vi "arm control.vi"(1 "State":T1, 2 "Z Axis (Tuning)":dbl) -> (0 "setpoint":dbl format="%.2f")   [LabVIEW 2013]
uses:
  typedefs/subStates.ctl
  typedefs/fg_typedef.ctl
panel:
  in  "lower limit":dbl=-0.015 format="%#_13g"
  in  "upper limit":dbl=0.015 format="%#_13g"
  in  "Up Setpoint":dbl format="%#_13g"
  # "Things needing Tuning"
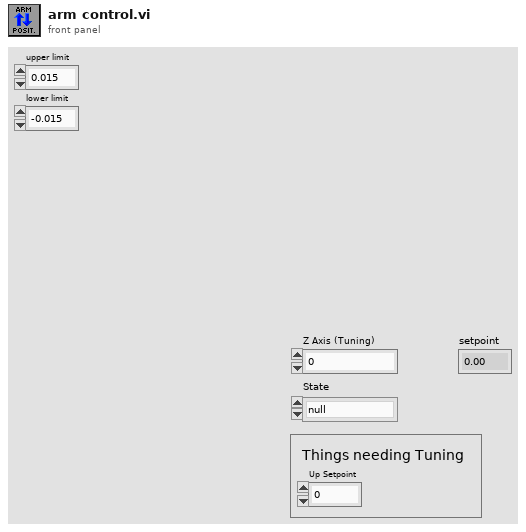
[diagram p1: front panel]
types:
  T1 = typedef "subStates.ctl" = enum16{"null", "wait", "driver control", "auto", "manual override", "hold position", "rotate", "pickup", "pass", "load", "goto shoot", "shoot", "cancel", "end"}
  T2 = typedef "fg_typedef.ctl" = enum16{"Get", "Set"}
  T3 = typedef "WPI_DigitalInputDevRef.ctl" = cluster{"DevStatus":errorcluster, "DIO Channel":T4, "Digital Module":T5}
  T4 = typedef "FPGA_DIOChannel.ctl" = enum8{"DIO 1", "DIO 2", "DIO 3", "DIO 4", "DIO 5", "DIO 6", "DIO 7", "DIO 8", "DIO 9", "DIO 10", "DIO 11", "DIO 12", "DIO 13", "DIO 14", "Invalid"}
  T5 = typedef "FPGA_TypedefDigitalModule.ctl" = enum16{"Digital Module 1", "Digital Module 2"}
  T6 = typedef "WPI_EncoderDevRef.ctl" = cluster{"DevStatus":errorcluster, "EncoderIndex":T7, "CounterIndex":T8, "DistancePerCount":dbl, "Decoding Type":T9}
  T7 = typedef "FPGA_EncoderIdx.ctl" = enum8{"Enc 0", "Enc 1", "Enc 2", "Enc 3", "Invalid"}
  T8 = typedef "FPGA_CounterCtrSystemIndex.ctl" = enum8{"Ctr 0", "Ctr 1", "Ctr 2", "Ctr 3", "Ctr 4", "Ctr 5", "Ctr 6", "Ctr 7", "Invalid"}
  T9 = typedef "WPI_EncoderType.ctl" = enum16{"1x", "2x", "4x"}
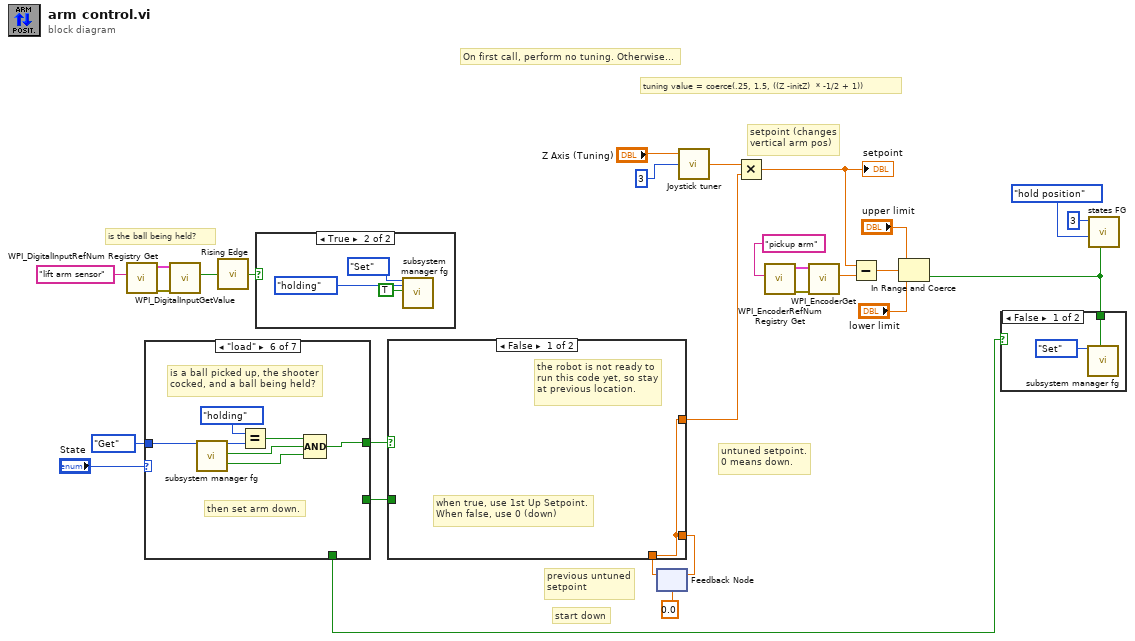
[diagram p0: block diagram]
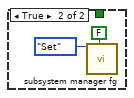
[diagram p2: hidden frame]
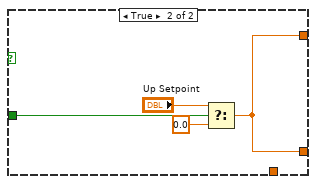
[diagram p4: hidden frame]
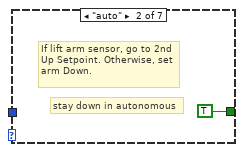
[diagram p6: hidden frame]
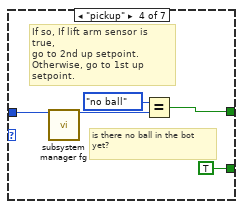
[diagram p8: hidden frame]
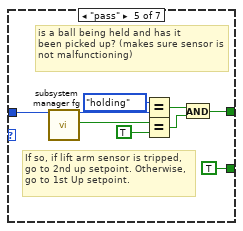
[diagram p9: hidden frame]
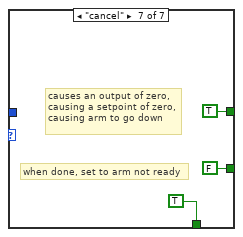
[diagram p10: hidden frame]
diagram:
  # "untuned setpoint.\n0 means down."
  # "tuning value = coerce(.25, 1.5, ((Z -initZ)  * -1/2 + 1))"
  # "On first call, perform no tuning. Otherwise..."
  # "is the ball being held?"
  # "start down"
  # "previous untuned\nsetpoint"
  # "setpoint (changes\nvertical arm pos)"
  n1 = call <vilib>:"WPI_DigitalInputRefNum Registry Get.vi"("refnum name"="lift arm sensor") -> ("error out"=w5:errorcluster, "DigitalInputDevRef"=w6:T3)  [unwired: 9 in]
  n2 = case shown="\"load\"" "State" {
    tunnel: fg_typedef."Get" ("Menu") -> [_ _ _ w34 w43 w50 _]
    tunnel: [_ TRUE _ w33 w38 w49 TRUE] -> w19
    tunnel: [_ _ _ TRUE ("y") TRUE ("y") _ FALSE ("y")] -> w18
    tunnel: [_ _ _ _ _ _ TRUE] -> w1
    frame "driver control", Default {
      # "code does not run"
    }
    frame "auto" {
      # "If lift arm sensor, go to 2nd\nUp Setpoint. Otherwise, set\narm Down."
      # "stay down in autonomous"
    }
    frame "manual override" {
      # "code does not run"
    }
    frame "pickup" {
      # "If so, If lift arm sensor is true,\ngo to 2nd up setpoint.\nOtherwise, go to 1st up\nsetpoint."
      # "is there no ball in the bot\nyet?"
      n3 = call "subsystem manager fg.vi"("Menu"=w34) -> ("Ball State Read"=w31:enum16{"no ball", "holding", "loaded"})  [unwired: 14 in, 4 out]
      n4 = Equal?(x=enum16{"no ball", "holding", "loaded"}."no ball" ("y"), y=w31) -> (x = y?=w33:bool)
    }
    frame "pass" {
      # "If so, if lift arm sensor is tripped,\ngo to 2nd up setpoint. Otherwise,\ngo to 1st Up setpoint."
      # "is a ball being held and has it\nbeen picked up? (makes sure sensor is\nnot malfunctioning)"
      n5 = call "subsystem manager fg.vi"("Menu"=w43) -> ("Ball State Read"=w36:enum16{"no ball", "holding", "loaded"}, "Picked Up"=w42:bool)  [unwired: 14 in, 3 out]
      n6 = Equal?(x=enum16{"no ball", "holding", "loaded"}."holding" ("y"), y=w36) -> (x = y?=w39:bool)
      n7 = Equal?(x=w42, y=TRUE) -> (x = y?=w40:bool)
      n8 = And(x=w39, y=w40) -> (x .and. y?=w38:bool)
    }
    frame "load" {
      # "then set arm down."
      # "is a ball picked up, the shooter\ncocked, and a ball being held?"
      n9 = call "subsystem manager fg.vi"("Menu"=w50) -> ("Ball State Read"=w48:enum16{"no ball", "holding", "loaded"}, "Picked Up"=w45:bool, "Shooter Cocked"=w44:bool)  [unwired: 14 in, 2 out]
      n10 = Equal?(x=enum16{"no ball", "holding", "loaded"}."holding", y=w48) -> (x = y?=w46:bool)
      n11 = Compound Arithmetic op=AND(w46, w45, w44) -> (w49:bool)
    }
    frame "cancel" {
      # "when done, set to arm not ready"
      # "causes an output of zero,\ncausing a setpoint of zero,\ncausing arm to go down"
    }
  }
  n12 = call <vilib>:"WPI_DigitalInputGetValue.vi"("error in (no error)"=w5, "DigitalInputDevRef"=w6) -> ("Value"=w8:bool)  [unwired: 7 in, 2 out]
  n13 = call "Rising Edge.vi"("Input"=w8) -> ("Rising Edge"=w9:bool)
  n14 = case shown="True" w9 {
    frame False {
    }
    frame True {
      n15 = call "subsystem manager fg.vi"("Menu"=fg_typedef."Set", "Ball State Write"=enum16{"no ball", "holding", "loaded"}."holding", "Picked Up"=TRUE) -> ()  [unwired: 12 in, 5 out]
    }
  }
  n16 = feedback #1(0.0 ("x")) -> (w11:dbl)
  n17 = case shown="False" w19 {
    tunnel: w18 -> [_ w59]
    tunnel: [w57 w58] -> w13
    tunnel: [w57 w58] -> w12
    tunnel: w11 -> [w57 _]
    frame False {
      # "when true, use 1st Up Setpoint.\nWhen false, use 0 (down)"
      # "the robot is not ready to\nrun this code yet, so stay\nat previous location."
    }
    frame True {
      n18 = Select(t="Up Setpoint", s=w59, f=0.0 ("x")) -> (s? t:f=w58:dbl)
    }
  }
  n19 = feedback-in #1(w12) -> ()
  n20 = call "Joystick tuner.vi"("Joystick Z"="Z Axis (Tuning)", "Loop ID"=3) -> ("Output"=w4:dbl)  [unwired: 7 in]
  n21 = Multiply(x=w4, y=w13) -> (x*y=w17:dbl)
  "setpoint" <- w17
  n22 = call <vilib>:"WPI_EncoderRefNum Registry Get.vi"("refnum name"="pickup arm") -> ("error out"=w22:errorcluster, "EncoderDevRef"=w23:T6)  [unwired: 9 in]
  n23 = call <vilib>:"WPI_EncoderGet.vi"("error in (no error)"=w22, "EncoderDevRef"=w23) -> ("Distance"=w28:dbl)  [unwired: 4 in, 5 out]
  n24 = Subtract(x=w17, y=w28) -> (x-y=w25:dbl)
  n25 = In Range and Coerce(upper limit="upper limit", x=w25, lower limit="lower limit") -> (In Range?=w15:bool)  [unwired: 1 out]
  n26 = case shown="False" w1 {
    tunnel: w15 -> [w62 _]
    frame False {
      n27 = call "subsystem manager fg.vi"("Menu"=fg_typedef."Set", "Arm Ready"=w62) -> ()  [unwired: 13 in, 5 out]
    }
    frame True {
      n28 = call "subsystem manager fg.vi"("Menu"=fg_typedef."Set", "Arm Ready"=FALSE) -> ()  [unwired: 13 in, 5 out]
    }
  }
  n29 = call "states FG.vi"("exit in"=w15, "subState in"=subStates."hold position", "Loop ID"=3) -> ()  [unwired: 5 in, 4 out]
